vi "WriteTreeToRCMFile.vi"(7 "tree control":refnum<class "TreeControl.lvclass">, 8 "error in (no error)":errorcluster, 11 "rcm file path in":path) -> (0 "error out":errorcluster, 3 "rcm file path out":path)   [LabVIEW 2020]
uses:
  Support/Tree Control/Library/TreeControl.lvclass
  Support/MSXML/Public/Type Definition/Attribute__slk_msxml.ctl
  Support/MSXML/Public/MSXML Document/msxml document.lvclass
  Support/MSXML/Library/MSXML.lvlib
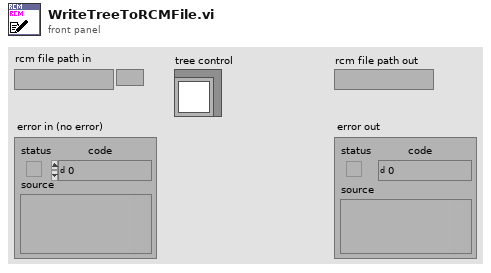
[diagram p1: front panel]
types:
  T1 = typedef "MSXML.lvlib/Attribute__slk_msxml.ctl" = cluster{"name":string, "value":string}
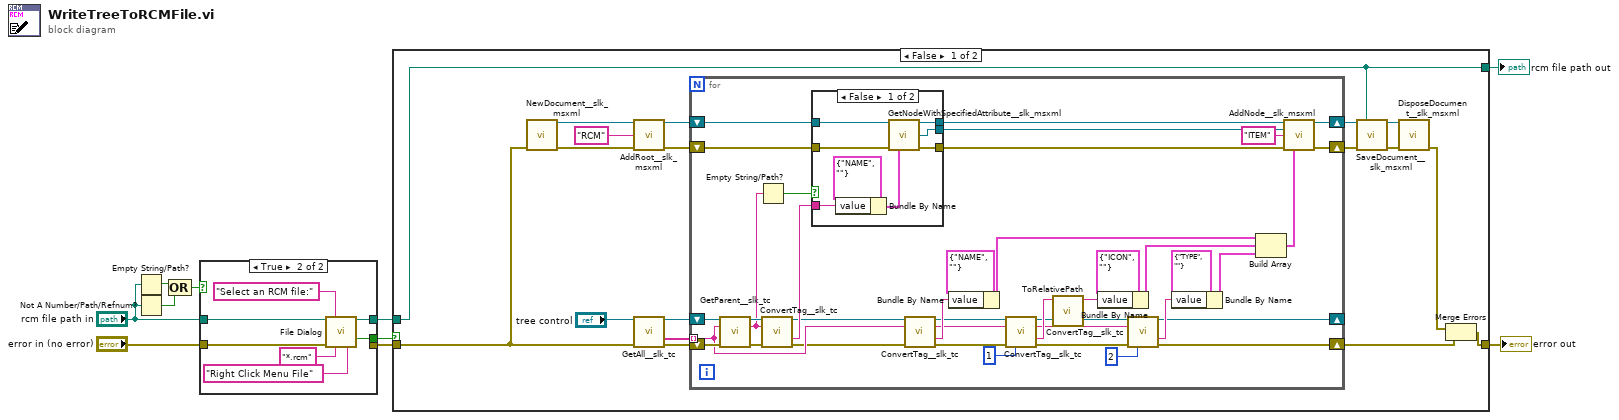
[diagram p0: block diagram]
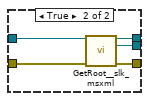
[diagram p2: hidden frame]
diagram:
  n1 = Empty String/Path?(string/path="rcm file path in") -> (empty?=w8:bool)
  n2 = Not A Number/Path/Refnum?(number/path/refnum="rcm file path in") -> (NaN/Path/Refnum?=w10:bool)
  n3 = Compound Arithmetic op=OR(w8, w10) -> (w4:bool)
  n4 = case shown="True" w4 {
    tunnel: "rcm file path in" -> [w12 w16]
    tunnel: [w12 w15] -> w7
    tunnel: [w11 _] -> w1
    tunnel: [_ w14] -> w9
    tunnel: "error in (no error)" -> [w11 w13]
    frame False {
    }
    frame True {
      n5 = call "File Dialog"("start path"=w16, "prompt"="Select an RCM file:", "error in"=w13, "pattern (all files)"="*.rcm", "pattern label"="Right Click Menu File") -> ("selected path"=w15:path, "cancelled"=w14:bool)  [unwired: 7 in, 2 out]
    }
  }
  n6 = case shown="False" w9 {
    tunnel: w1 -> [w22 w91]
    tunnel: w7 -> [w20 w90]
    tunnel: [w21 w91] -> w3
    tunnel: [w20 w90] -> w2
    frame False {
      n7 = call "NewDocument__slk_msxml.vi"("error in (no error)"=w22) -> ("document out"=w27:refnum<class "msxml document.lvclass">, "error out"=w26:errorcluster)  [unwired: 13 in]
      n8 = call "AddRoot__slk_msxml.vi"("document in"=w27, "node name"="RCM", "error in (no error)"=w26) -> ("document out"=w33:refnum<class "msxml document.lvclass">, "error out"=w31:errorcluster)  [unwired: 10 in, 1 out]
      n9 = call "GetAll__slk_tc.vi"("tree control in"="tree control", "error in (no error)"=w22) -> ("tree control out"=w36:refnum<class "TreeControl.lvclass">, "output tree items"=w34:string[], "error out"=w35:errorcluster)  [unwired: 10 in, 1 out]
      n10 = for {
        shift-right: [w52] -> w23
        shift-left: w35 -> [w75]
        shift-right: [w45] -> _
        shift-left: w36 -> [w76]
        tunnel: w34 -> [w65] mode=indexing
        shift-right: [w69] -> w30
        shift-left: w33 -> [w74]
        shift-right: [w68] -> w29
        shift-left: w31 -> [w72]
        n11 = call "GetParent__slk_tc.vi"("tree control in"=w76, "child tag (\"\")"=w65, "error in (no error)"=w75) -> ("tree control out"=w44:refnum<class "TreeControl.lvclass">, "parent tag"=w41:string, "error out"=w42:errorcluster)  [unwired: 9 in, 1 out]
        n12 = Empty String/Path?(string/path=w41) -> (empty?=w73:bool)
        n13 = call "ConvertTag__slk_tc.vi"("tree control in"=w44, "input tag (current tag)"=w41, "error in (no error)"=w42) -> ("tree control out"=w39:refnum<class "TreeControl.lvclass">, "text"=w43:string, "error out"=w40:errorcluster)  [unwired: 9 in, 1 out]
        n14 = case shown="False" w73 {
          tunnel: w74 -> [w84 w89]
          tunnel: [w83 w88] -> w70
          tunnel: [w82 w87] -> w71
          tunnel: [w81 w86] -> w66
          tunnel: w72 -> [w80 w85]
          tunnel: w43 -> [w77 _]
          frame False {
            n15 = Bundle By Name(cluster=T1 {"name"="NAME", "value"=""} ("attribute"), "value"=w77) -> (w78:T1)
            n16 = call "GetNodeWithSpecifiedAttribute__slk_msxml.vi"("document in"=w84, "error in (no error)"=w80, "attribute"=w78) -> ("document out"=w82:refnum<class "msxml document.lvclass">, "first node out"=w81:refnum<class "msxml node.lvclass">, "error out"=w83:errorcluster)  [unwired: 9 in, 1 out]
          }
          frame True {
            n17 = call "GetRoot__slk_msxml.vi"("document in"=w89, "error in (no error)"=w85) -> ("document out"=w87:refnum<class "msxml document.lvclass">, "root node out"=w86:refnum<class "msxml node.lvclass">, "error out"=w88:errorcluster)  [unwired: 11 in]
          }
        }
        n18 = call "ConvertTag__slk_tc.vi"("tree control in"=w39, "input tag (current tag)"=w65, "error in (no error)"=w40) -> ("tree control out"=w61:refnum<class "TreeControl.lvclass">, "duplicated tag"=w60:string, "text"=w64:string, "error out"=w59:errorcluster)  [unwired: 9 in]
        n19 = Bundle By Name(cluster=T1 {"name"="NAME", "value"=""} ("attribute"), "value"=w64) -> (w46:T1)
        n20 = call "ConvertTag__slk_tc.vi"("tree control in"=w61, "input tag (current tag)"=w60, "error in (no error)"=w59, "column # (0)"=1) -> ("tree control out"=w55:refnum<class "TreeControl.lvclass">, "duplicated tag"=w54:string, "text"=w63:string, "error out"=w53:errorcluster)  [unwired: 8 in]
        n21 = call "ToRelativePath.vi"("absolutely path"=w63) -> ("relative path"=w38:string)  [unwired: 10 in]
        n22 = Bundle By Name(cluster=T1 {"name"="ICON", "value"=""} ("attribute"), "value"=w38) -> (w48:T1)
        n23 = call "ConvertTag__slk_tc.vi"("tree control in"=w55, "input tag (current tag)"=w54, "error in (no error)"=w53, "column # (0)"=2) -> ("tree control out"=w45:refnum<class "TreeControl.lvclass">, "text"=w56:string, "error out"=w52:errorcluster)  [unwired: 8 in, 1 out]
        n24 = Bundle By Name(cluster=T1 {"name"="TYPE", "value"=""} ("attribute"), "value"=w56) -> (w47:T1)
        n25 = Build Array(w46, w48, w47) -> (w50:T1[])
        n26 = call "AddNode__slk_msxml.vi"("document in"=w71, "parent node in"=w66, "node name"="ITEM", "error in (no error)"=w70, "attributes"=w50) -> ("document out"=w69:refnum<class "msxml document.lvclass">, "error out"=w68:errorcluster)  [unwired: 8 in, 1 out]
      }
      n27 = call "SaveDocument__slk_msxml.vi"("document in"=w30, "xml document path in"=w20, "error in (no error)"=w29) -> ("document out"=w28:refnum<class "msxml document.lvclass">, "error out"=w25:errorcluster)  [unwired: 11 in]
      n28 = call "DisposeDocument__slk_msxml.vi"("document in"=w28, "error in (no error)"=w25) -> ("error out"=w24:errorcluster)  [unwired: 13 in]
      n29 = Merge Errors(w24, w23) -> (w21:errorcluster)
    }
    frame True {
    }
  }
  "error out" <- w3
  "rcm file path out" <- w2
